vi "Initialize.vi"(8 "error in (no error)":errorcluster, 11 "dir":string) -> (0 "error out":errorcluster, 2 "function return":u32, 3 "dir out":string)   [LabVIEW 2014, in "atmcd32d.lvlib"]
doc: "unsigned int WINAPI Initialize(char * dir);"
uses:
  atmcd32d.lvlib
  atmcd32d.dll
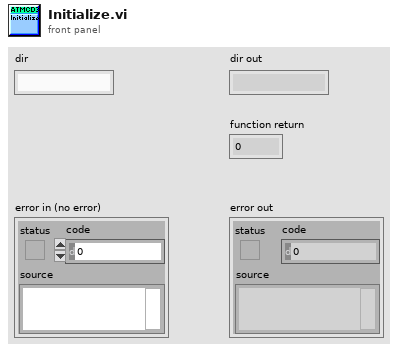
[diagram p1: front panel]
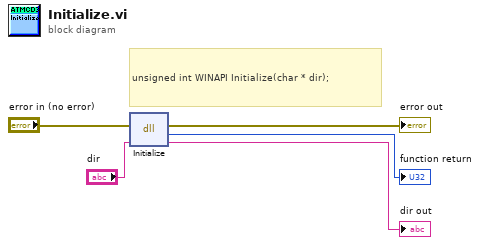
[diagram p0: block diagram]
diagram:
  # "unsigned int WINAPI Initialize(char * dir);"
  n1 = dll-call lib="C:/Users/Bakir/Documents/Lambda2-Testing/lib/Andorlib/atmcd32d.*" fn="Initialize"(error in="error in (no error)", "dir"="dir") -> (error out=→"error out":errorcluster, →"function return":u32, "dir"=→"dir out":string)  [unwired: 2 in, 1 out]
